vi "minicryo_T-control.vi"(5 "Ramp Mode":bool, 7 "Rate  [K/min]":dbl=0.1, 9 "VISA resource name out":refnum<visa-resource-name>="COM7", 11 "Set Sample Temp [K]":dbl=1.5) -> ()   [LabVIEW 2013]
panel:
  in  "Heater":bool
  out "String":string="+023.261E+0;+022.689E+0\n"
  in  "Auto PID":bool=TRUE
  out "D2":string="0"
  out "I2":string="10.095924"
  out "P2":string="150"
  out "D1":string="0"
  out "I1":string="40"
  out "P1":string="120"
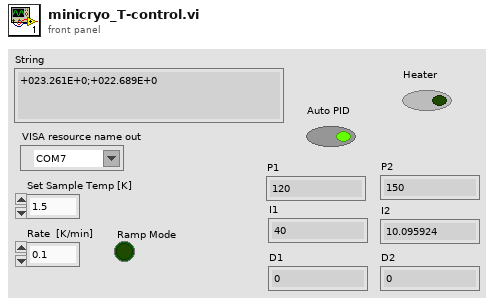
[diagram p1: front panel]
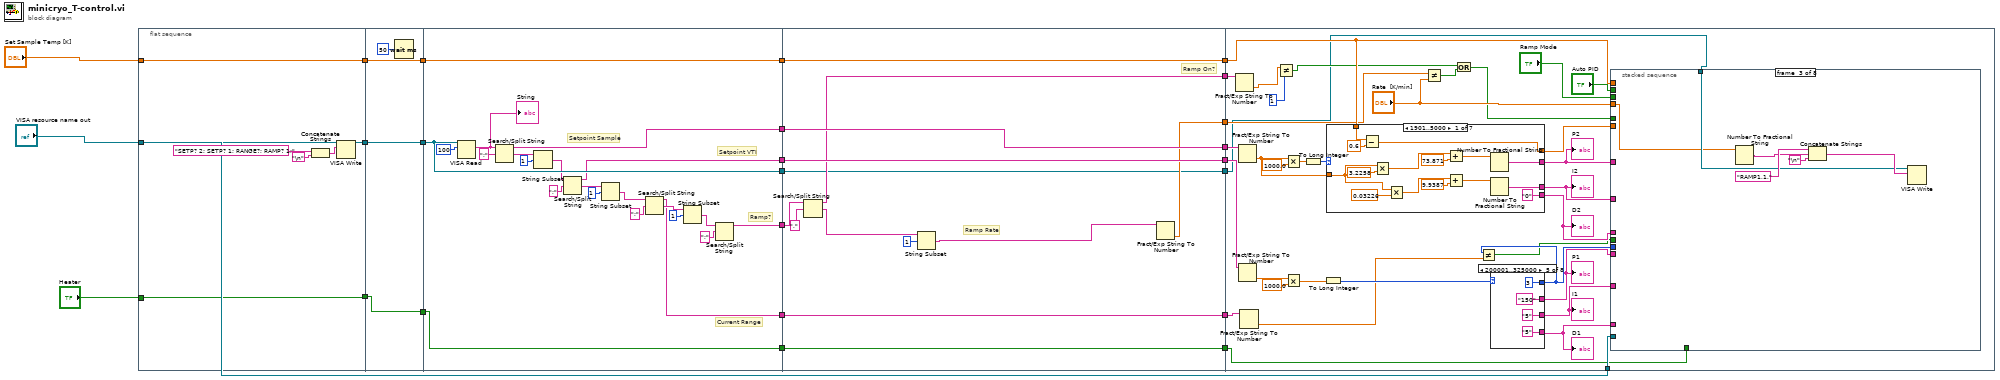
[diagram p0: block diagram]
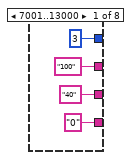
[diagram p2: hidden frame]
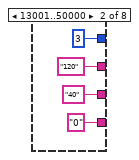
[diagram p3: hidden frame]
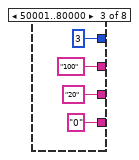
[diagram p4: hidden frame]
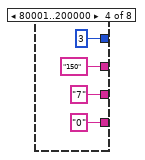
[diagram p5: hidden frame]
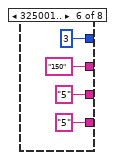
[diagram p6: hidden frame]
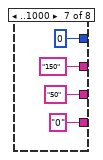
[diagram p7: hidden frame]
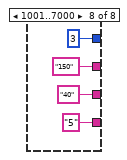
[diagram p8: hidden frame]
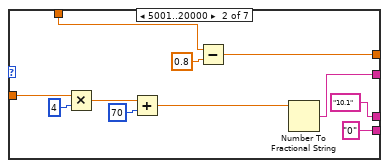
[diagram p9: hidden frame]
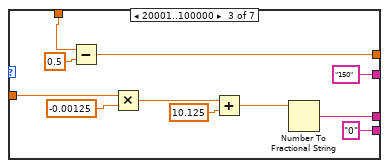
[diagram p10: hidden frame]
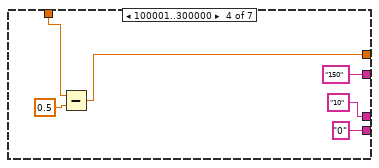
[diagram p11: hidden frame]
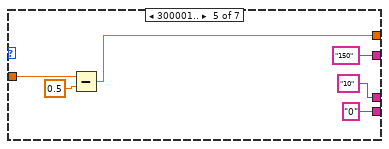
[diagram p12: hidden frame]
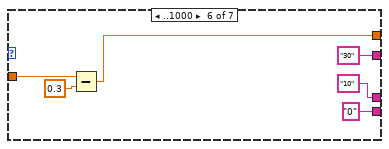
[diagram p13: hidden frame]
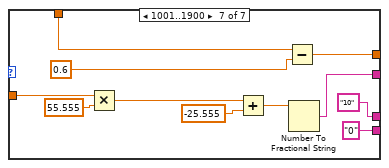
[diagram p14: hidden frame]
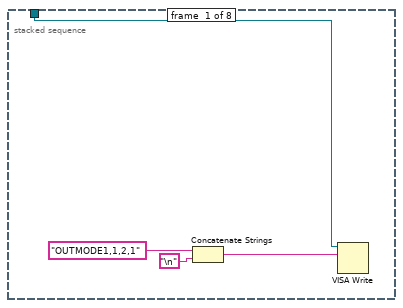
[diagram p15: hidden frame]
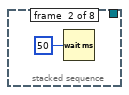
[diagram p16: hidden frame]
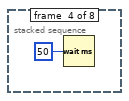
[diagram p17: hidden frame]
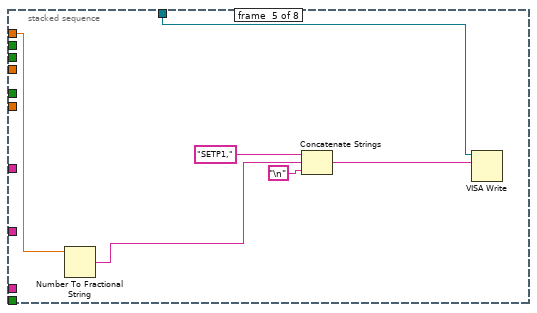
[diagram p18: hidden frame]
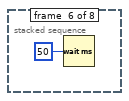
[diagram p19: hidden frame]
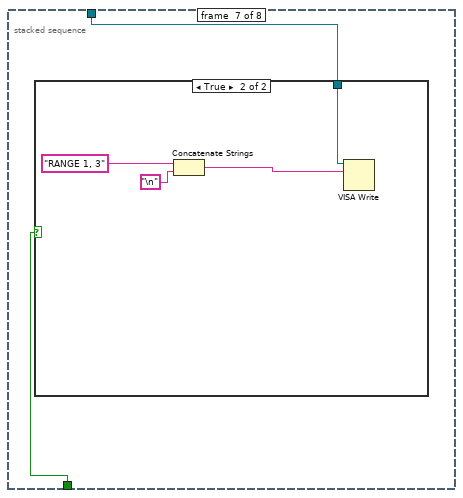
[diagram p20: hidden frame]
diagram:
  n1 = flat-sequence {
    tunnel: "VISA resource name out" -> [w27]
    tunnel: "Set Sample Temp [K]" -> [w31]
    tunnel: [w31] -> w17
    tunnel: [w26] -> w16
    tunnel: [w25] -> w5
    tunnel: "Heater" -> [w25]
    tunnel: [w35] -> w19
    tunnel: [w34] -> w18
    tunnel: w17 -> [w35]
    tunnel: w16 -> [w34]
    tunnel: w5 -> [w32]
    tunnel: [w32] -> w3
    tunnel: [w57] -> w21
    tunnel: [w55] -> w20
    tunnel: w19 -> [w57]
    tunnel: w18 -> [w55]
    tunnel: [w51] -> w15
    tunnel: [w45] -> w14
    tunnel: [w39] -> w10
    tunnel: [w37] -> w9
    tunnel: w3 -> [w36]
    tunnel: [w36] -> w2
    tunnel: [w70] -> w22
    tunnel: [w69] -> w13
    tunnel: [w68] -> w12
    tunnel: [w67] -> w11
    tunnel: w21 -> [w70]
    tunnel: w20 -> [w59]
    tunnel: w15 -> [w68]
    tunnel: w14 -> [w69]
    tunnel: w10 -> [w67]
    tunnel: w9 -> [w66]
    tunnel: [w64] -> w8
    tunnel: [w60] -> w7
    tunnel: [w59] -> w6
    tunnel: w2 -> [w58]
    tunnel: [w58] -> w1
    tunnel: "VISA resource name out" -> [w91]
    tunnel: w22 -> [w85]
    tunnel: w13 -> [w89]
    tunnel: w12 -> [w87]
    tunnel: w11 -> [w84]
    tunnel: w8 -> [w80]
    tunnel: w7 -> [w76]
    tunnel: w6 -> [w72]
    tunnel: w1 -> [w71]
    frame #0 {
      n2 = Concatenate Strings("SETP? 2; SETP? 1; RANGE?; RAMP? 1;" ("write buffer"), "\n") -> (w28:string)
      n3 = VISA Write(VISA resource name=w27, write buffer=w28) -> (VISA resource name out=w26:refnum<visa-resource-name>)  [unwired: 1 in, 2 out]
    }
    frame #1 {
      n4 = Wait (ms)(milliseconds to wait=50) -> ()  [unwired: 1 out]
    }
    frame #2 {
      # "Ramp?"
      # "Current Range"
      # "Setpoint VTI"
      # "Setpoint Sample"
      n5 = VISA Read(VISA resource name=w55, byte count=u32 100) -> (read buffer=w50:string)  [unwired: 1 in, 3 out]
      "String" <- w50
      n6 = Search/Split String(string=w50, search string/char (-)=";") -> (substring before match=w51:string, match + rest of string=w53:string)  [unwired: 1 in, 1 out]
      n7 = String Subset(string=w53, offset (0)=u32 1 ("byte count")) -> (substring=w46:string)  [unwired: 1 in]
      n8 = Search/Split String(string=w46, search string/char (-)=";") -> (substring before match=w45:string, match + rest of string=w49:string)  [unwired: 1 in, 1 out]
      n9 = String Subset(string=w49, offset (0)=u32 1 ("byte count")) -> (substring=w40:string)  [unwired: 1 in]
      n10 = Search/Split String(string=w40, search string/char (-)=";") -> (substring before match=w39:string, match + rest of string=w44:string)  [unwired: 1 in, 1 out]
      n11 = String Subset(string=w44, offset (0)=u32 1 ("byte count")) -> (substring=w38:string)  [unwired: 1 in]
      n12 = Search/Split String(string=w38, search string/char (-)=";") -> (substring before match=w37:string)  [unwired: 1 in, 2 out]
    }
    frame #3 {
      # "Ramp Rate"
      # "Ramp On?"
      n13 = Search/Split String(string=w66, search string/char (-)=",") -> (substring before match=w64:string, match + rest of string=w62:string)  [unwired: 1 in, 1 out]
      n14 = String Subset(string=w62, offset (0)=u32 1 ("byte count")) -> (substring=w61:string)  [unwired: 1 in]
      n15 = Fract/Exp String To Number(string=w61) -> (number=w60:dbl)  [unwired: 3 in, 1 out]
    }
    frame #4 {
      n16 = Fract/Exp String To Number(string=w80) -> (number=w79:dbl)  [unwired: 3 in, 1 out]
      n17 = Fract/Exp String To Number(string=w87) -> (number=w86:dbl)  [unwired: 3 in, 1 out]
      n18 = Fract/Exp String To Number(string=w89) -> (number=w88:dbl)  [unwired: 3 in, 1 out]
      n19 = Fract/Exp String To Number(string=w84) -> (number=w83:dbl)  [unwired: 3 in, 1 out]
      n20 = Not Equal?(x=w79, y=1) -> (x != y?=w74:bool)
      n21 = Multiply(x=w86, y=1000.0) -> (x*y=w103:dbl)
      n22 = Multiply(x=w88, y=1000.0) -> (x*y=w100:dbl)
      n23 = To Long Integer(number=w103) -> (32bit integer=w104:i32)
      n24 = To Long Integer(number=w100) -> (32bit integer=w99:i32)
      n25 = case shown="1901..5000" w104 {
        tunnel: w86 -> [w140 w159 w169 _ w185 w191 w194]
        tunnel: [w146 w158 w168 w179 w184 w190 w200] -> w90
        tunnel: [w148 w157 "150" "150" "150" "30" w198] -> w95
        tunnel: [w139 "10.1" w166 "10" "10" "10" "10"] -> w94
        tunnel: ["0" "0" "0" "0" "0" "0" "0"] -> w93
        tunnel: w85 -> [w138 w153 w164 w175 _ _ w193]
        frame 1901..5000 {
          n26 = Subtract(x=w138, y=0.6) -> (x-y=w146:dbl)
          n27 = Multiply(x=w140, y=3.2258) -> (x*y=w150:dbl)
          n28 = Multiply(x=w140, y=0.03226) -> (x*y=w142:dbl)
          n29 = Add(x=w150, y=73.871) -> (x+y=w149:dbl)
          n30 = Add(x=w142, y=9.9387) -> (x+y=w141:dbl)
          n31 = Number To Fractional String(number=w149) -> (F-format string=w148:string)  [unwired: 3 in]
          n32 = Number To Fractional String(number=w141) -> (F-format string=w139:string)  [unwired: 3 in]
        }
        frame 5001..20000 {
          n33 = Multiply(x=w159, y=4) -> (x*y=w161:dbl)
          n34 = Add(x=w161, y=70) -> (x+y=w160:dbl)
          n35 = Subtract(x=w153, y=0.8) -> (x-y=w158:dbl)
          n36 = Number To Fractional String(number=w160) -> (F-format string=w157:string)  [unwired: 3 in]
        }
        frame 20001..100000 {
          n37 = Subtract(x=w164, y=0.5) -> (x-y=w168:dbl)
          n38 = Multiply(x=w169, y=-0.00125) -> (x*y=w172:dbl)
          n39 = Add(x=w172, y=10.125) -> (x+y=w171:dbl)
          n40 = Number To Fractional String(number=w171) -> (F-format string=w166:string)  [unwired: 3 in]
        }
        frame 100001..300000 {
          n41 = Subtract(x=w175, y=0.5) -> (x-y=w179:dbl)
        }
        frame 300001.. {
          n42 = Subtract(x=w185, y=0.5) -> (x-y=w184:dbl)
        }
        frame ..1000 {
          n43 = Subtract(x=w191, y=0.3) -> (x-y=w190:dbl)
        }
        frame 1001..1900 {
          n44 = Multiply(x=w194, y=55.555) -> (x*y=w201:dbl)
          n45 = Add(x=w201, y=-25.555) -> (x+y=w199:dbl)
          n46 = Subtract(x=w193, y=0.6) -> (x-y=w200:dbl)
          n47 = Number To Fractional String(number=w199) -> (F-format string=w198:string)  [unwired: 3 in]
        }
      }
      "P2" <- w95
      "I2" <- w94
      "D2" <- w93
      n48 = Not Equal?(x=w76, y="Rate  [K/min]") -> (x != y?=w75:bool)
      n49 = Or(x=w74, y=w75) -> (x .or. y?=w73:bool)
      n50 = case shown="200001..325000" w99 {
        tunnel: [3 3 3 3 3 3 0 3] -> w82
        tunnel: ["100" "120" "100" "150" "150" "150" "150" "150"] -> w98
        tunnel: ["40" "40" "20" "7" "5" "5" "50" "40"] -> w97
        tunnel: ["0" "0" "0" "0" "5" "5" "0" "5"] -> w96
        frame 7001..13000 {
        }
        frame 13001..50000 {
        }
        frame 50001..80000 {
        }
        frame 80001..200000 {
        }
        frame 200001..325000 {
        }
        frame 325001.. {
        }
        frame ..1000 {
        }
        frame 1001..7000 {
        }
      }
      "P1" <- w98
      "I1" <- w97
      "D1" <- w96
      n51 = Not Equal?(x=w82, y=w83) -> (x != y?=w81:bool)
      n52 = stacked-sequence {
        tunnel: w91 -> [_ _ _ _ _ _ _ _]
        tunnel: w90 -> [_ _ _ _ _ _ _ _]
        tunnel: "Rate  [K/min]" -> [_ _ w209 _ _ _ _ _]
        tunnel: w95 -> [_ _ _ _ _ _ _ _]
        tunnel: w94 -> [_ _ _ _ _ _ _ _]
        tunnel: w93 -> [_ _ _ _ _ _ _ _]
        tunnel: "Ramp Mode" -> [_ _ _ _ _ _ _ _]
        tunnel: w85 -> [_ _ _ _ w216 _ _ _]
        tunnel: w82 -> [_ _ _ _ _ _ _ _]
        tunnel: w98 -> [_ _ _ _ _ _ _ _]
        tunnel: w97 -> [_ _ _ _ _ _ _ _]
        tunnel: w96 -> [_ _ _ _ _ _ _ _]
        tunnel: "Auto PID" -> [_ _ _ _ _ _ _ _]
        tunnel: w81 -> [_ _ _ _ _ _ _ _]
        tunnel: w73 -> [_ _ _ _ _ _ _ _]
        tunnel: w72 -> [w204 _ w210 _ w217 _ w223 _]
        tunnel: w71 -> [_ _ _ _ _ _ w224 _]
        frame #0 {
          n53 = Concatenate Strings("OUTMODE1,1,2,1" ("write buffer"), "\n") -> (w205:string)
          n54 = VISA Write(VISA resource name=w204, write buffer=w205) -> ()  [unwired: 1 in, 3 out]
        }
        frame #1 {
          n55 = Wait (ms)(milliseconds to wait=u32 50) -> ()  [unwired: 1 out]
        }
        frame #2 {
          n56 = Number To Fractional String(number=w209) -> (F-format string=w211:string)  [unwired: 3 in]
          n57 = Concatenate Strings("RAMP1,1," ("write buffer"), w211, "\n") -> (w213:string)
          n58 = VISA Write(VISA resource name=w210, write buffer=w213) -> ()  [unwired: 1 in, 3 out]
        }
        frame #3 {
          n59 = Wait (ms)(milliseconds to wait=u32 50) -> ()  [unwired: 1 out]
        }
        frame #4 {
          n60 = Number To Fractional String(number=w216) -> (F-format string=w218:string)  [unwired: 3 in]
          n61 = Concatenate Strings("SETP1," ("write buffer"), w218, "\n") -> (w220:string)
          n62 = VISA Write(VISA resource name=w217, write buffer=w220) -> ()  [unwired: 1 in, 3 out]
        }
        frame #5 {
          n63 = Wait (ms)(milliseconds to wait=u32 50) -> ()  [unwired: 1 out]
        }
        frame #6 {
          n64 = case shown="True" w224 {
            tunnel: w223 -> [_ w225]
            frame False {
            }
            frame True {
              n65 = Concatenate Strings("RANGE 1, 3" ("write buffer"), "\n") -> (w228:string)
              n66 = VISA Write(VISA resource name=w225, write buffer=w228) -> ()  [unwired: 1 in, 3 out]
            }
          }
        }
        frame #7 {
          n67 = Wait (ms)(milliseconds to wait=u32 50) -> ()  [unwired: 1 out]
        }
      }
    }
  }
